vi "Check Time.vi"(8 "error in (no error)":errorcluster, 11 "Attributes in":refnum<class "Attributes.lvclass">) -> (0 "error out":errorcluster, 2 "Complete?":bool, 3 "Attributes out":refnum<class "Attributes.lvclass">)   [LabVIEW 2021, in "Attributes.lvclass"]
uses:
  Attributes.lvclass
  Attributes.lvclass/Attributes.ctl
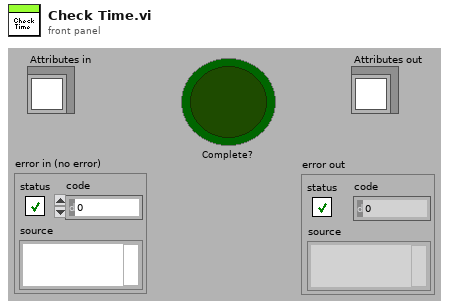
[diagram p1: front panel]
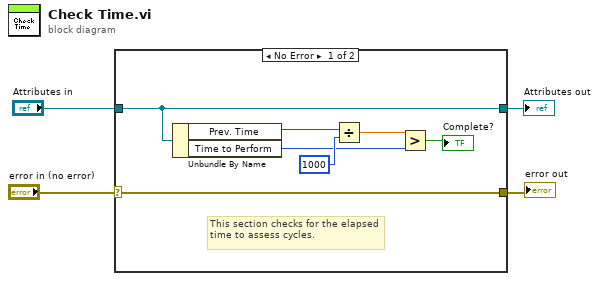
[diagram p0: block diagram]
diagram:
  n1 = case shown="No Error" "error in (no error)" {
    selector: "error in (no error)" -> [w11 w13]
    tunnel: [w11 w13] -> w3
    tunnel: [w10 w12] -> w1
    tunnel: "Attributes in" -> [w10 w12]
    frame No Error {
      # "This section checks for the elapsed time to assess cycles."
      n2 = Unbundle By Name(w10) -> ("Prev. Time"=w8:u32, "Time to Perform"=w6:u32)
      n3 = Divide(x=w8, y=u32 1000) -> (x/y=w5:dbl)
      n4 = Greater?(x=w5, y=w6) -> (0:→"Complete?":bool)
    }
    frame Error {
    }
  }
  "error out" <- w3
  "Attributes out" <- w1
